vi "Query SESR.vi"(8 "error in (no error)":errorcluster {"code" format="%.0x"}, 11 "VISA session":refnum<visa-resource-name>) -> (0 "error out":errorcluster {"code" format="%.0x"}, 1 "Read SESR":T1, 3 "dup VISA session":refnum<visa-resource-name>)   [LabVIEW 2011]
doc: "Reads the instrument's IEEE-488.2 Standard Event Status Register.\n\nThe bits in the event register are cleared automatically after calling this VI.\n\nNote: Do not call this VI between a VISA Write sending an instrument query and the corresponding VISA Read that retrieves the response. Doing so is likely to result in a query error on your instrument.\n\nNotes: \n(1) The error out is not modified if the Standard Event results indicates an instrument error occurred. Use the Query SESR for Instrument Error.vi if you want to the error out to reflect instrument error conditions.\n(2) Calling this VI clears the contents of the Standard Event Status Register."
uses:
  Low Level/Standard Event Status Indicator.ctl
panel:
  # "standard event status register (SESR)"
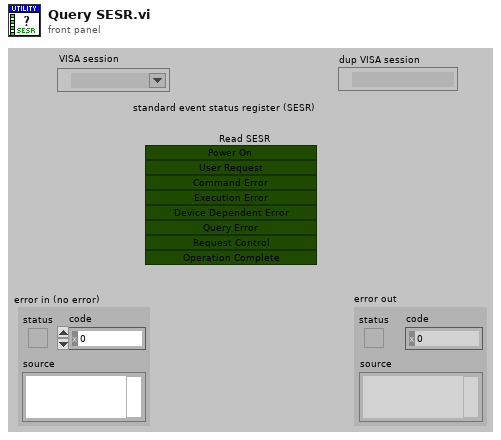
[diagram p1: front panel]
types:
  T1 = typedef "Standard Event Status Indicator.ctl" = cluster{"Operation Complete (1)":bool, "Request Control (2)":bool, "Query Error (4)":bool, "Device Dependent Error (8)":bool, "Execution Error (16)":bool, "Command Error (32)":bool, "User Request (64)":bool, "Power On (128)":bool}
  T2 = cluster{"[0]":bool, "[1]":bool, "[2]":bool, "[3]":bool, "[4]":bool, "[5]":bool, "[6]":bool, "[7]":bool}
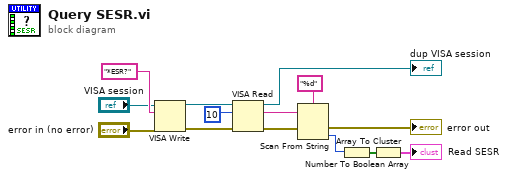
[diagram p0: block diagram]
diagram:
  n1 = VISA Write(VISA resource name="VISA session", write buffer="*ESR?", error in (no error)="error in (no error)") -> (VISA resource name out=w12:refnum<visa-resource-name>, error out=w13:errorcluster)  [unwired: 1 out]
  n2 = VISA Read(VISA resource name=w12, byte count=10, error in (no error)=w13) -> (VISA resource name out=→"dup VISA session":refnum<visa-resource-name>, read buffer=w10:string, error out=w3:errorcluster)  [unwired: 1 out]
  n3 = Scan From String(format string="%d", input string=w10, error in=w3) -> (error out=→"error out":errorcluster, output 1=w4:i32)  [unwired: 2 in, 2 out]
  n4 = Number To Boolean Array(number=w4) -> (Boolean array=w14:bool[])
  n5 = Array To Cluster(array=w14) -> (cluster=→"Read SESR":T2)
